vi "InStrSuchen_PossibleBug.vi"() -> ()   [LabVIEW 2014]
panel:
  out "Ausgang 1":bool
  out "Fehler (Ausgang)":errorcluster
  in  "Fehler (Eingang)":errorcluster
  out "Verbleibender String":string
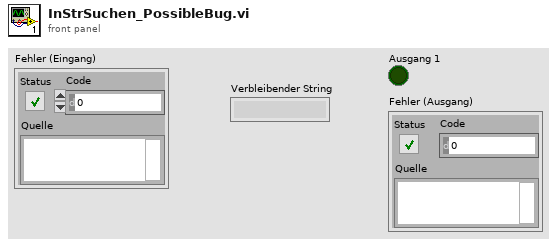
[diagram p1: front panel]
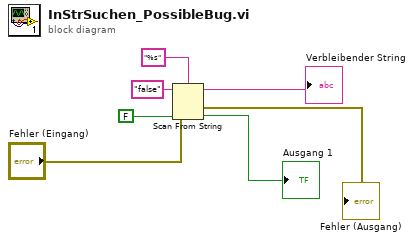
[diagram p0: block diagram]
diagram:
  n1 = Scan From String(format string="%s" ("Format-String"), input string="false" ("Eingangs-String"), error in="Fehler (Eingang)", default 1=FALSE) -> (remaining string=→"Verbleibender String":string, error out=→"Fehler (Ausgang)":errorcluster, output 1=→"Ausgang 1":bool)  [unwired: 1 in, 1 out]
